vi "set Frame Size LV.vi"(5 "vbin":i32, 6 "hbin":i32, 7 "vend":i32, 8 "error in (no error)":errorcluster, 9 "vstart":i32, 10 "hend":i32, 11 "hstart":i32) -> (0 "error out":errorcluster)   [LabVIEW 2016, in "cameraLibrary.lvlib"]
doc: "Set the frame size for sub-window acquisition.\n\n\n\nvoid CAMERALIBRARYSHARED_EXPORT setFrameSizeLV(int hstart, int hend, int vstart, int vend, int hbin, int vbin);"
uses:
  cameraLibrary.lvlib
  cameraLibrary.dll
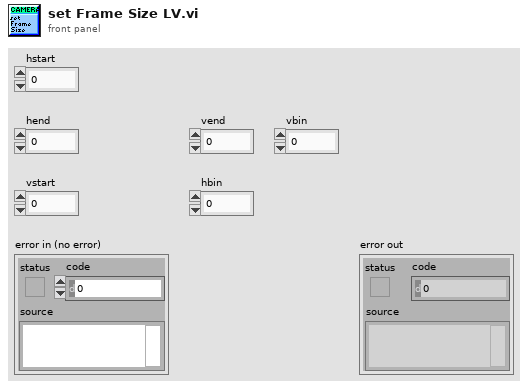
[diagram p1: front panel]
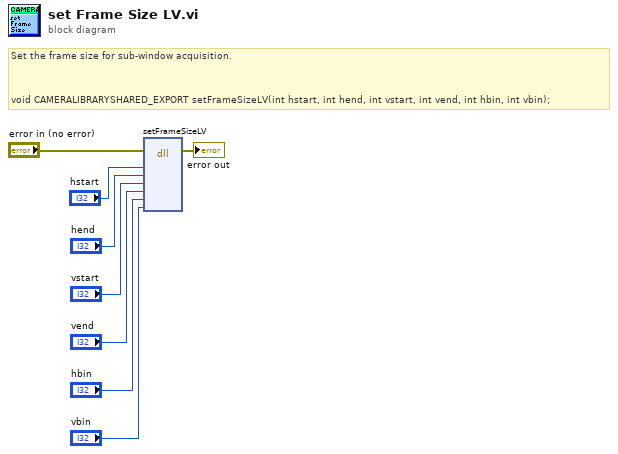
[diagram p0: block diagram]
diagram:
  # "Set the frame size for sub-window acquisition.\n\n\n\nvoid CAMERALIBRARYSHARED_EXPORT setFrameSizeLV(int hstart, int hend, int vstart, int vend, int hbin, int vbin);"
  n1 = dll-call lib="C:/Users/TMM/repos/EXPRES/FEM/FTT/support/Camera Library/cameraLibrary.*" fn="setFrameSizeLV"(error in="error in (no error)", "hstart"="hstart", "hend"="hend", "vstart"="vstart", "vend"="vend", "hbin"="hbin", "vbin"="vbin") -> (error out=→"error out":errorcluster)  [unwired: 9 in, 1 out]
